vi "Simple Reader.vi"(8 "error in (no error)":errorcluster, 11 "HP Counter Driver in":refnum<class "HP Counter Driver.lvclass">) -> (0 "error out":errorcluster, 2 "Signals":dbl[](array[numeric]), 3 "HP Counter Driver out":refnum<class "HP Counter Driver.lvclass">)   [LabVIEW 2019, in "HP Counter Driver.lvclass"]
uses:
  HP Counter Driver.lvclass
  C:/GitHub/NHMFL_Core/Libraries/Instruments/VISA Instrument/VISA Instrument.lvclass
  VISA Instrument/VISA Instrument.lvclass/VISA Instrument.ctl
  VISA Instrument/Read VISA resource.vi
  VISA Instrument/Write VISA resource.vi
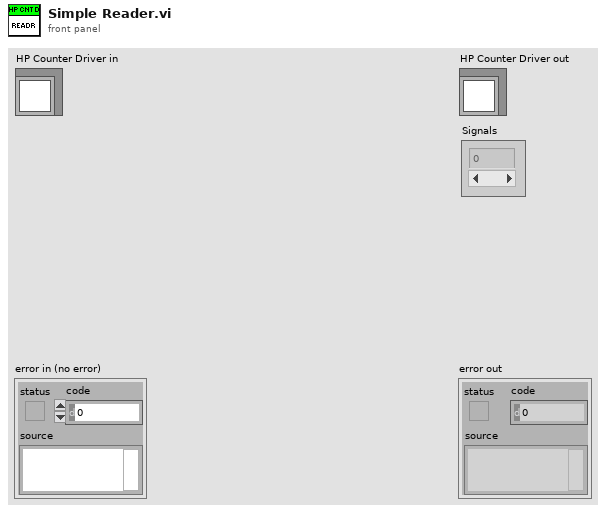
[diagram p1: front panel]
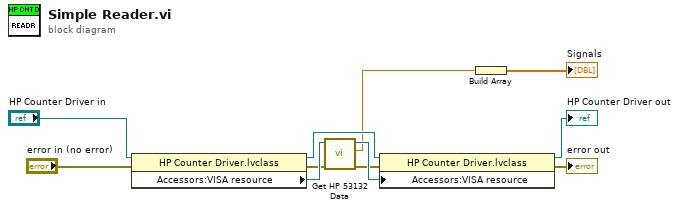
[diagram p0: block diagram]
diagram:
  n1 = property class="HP Counter Driver.lvclass"(reference="HP Counter Driver in", error in="error in (no error)") -> (reference out=w9:refnum<class "HP Counter Driver.lvclass">, error out=w4:errorcluster, "Accessors:VISA resource"=w6:refnum<visa-resource-name>)
  n2 = call "Get HP 53132 Data.vi"("error in (no error)"=w4, "VISA Resource Name"=w6) -> ("error out"=w3:errorcluster, "Data"=w2:dbl, "VISA Resource Name Out"=w5:refnum<visa-resource-name>)  [unwired: 6 in]
  n3 = property class="HP Counter Driver.lvclass"(reference=w9, error in=w3, "Accessors:VISA resource"=w5) -> (reference out=→"HP Counter Driver out":refnum<class "HP Counter Driver.lvclass">, error out=→"error out":errorcluster)
  n4 = Build Array(w2) -> (→"Signals":dbl[])
